vi "S4GUI.vi"(7 "Tab ObsEng":enum32{"Obs", "CCD modes", "Eng"}(tab)) -> ()   [LabVIEW 2018] (continued)
                    n457 = property on="setupCH4" class="Bool (strict)"("Blinking"=w1016) -> ()  [unwired: 2 in, 2 out]
                    n458 = property on="Disk Storage ch4" class="Slide (strict)"("Fill Color"=w1006) -> ()  [unwired: 2 in, 2 out]
                    n459 = Select(t=w1004, s=w1002, f=w1005) -> (s? t:f=w1003:cluster{u32, u32}[])
                    n460 = property on="Exposures Done ch4" class="Slide (strict)"("Caption.Text"=w1011) -> ()  [unwired: 2 in, 2 out]
                    n461 = property on="Channel 4" class="Bool (strict)"("Colors [4]"=w1003) -> ()  [unwired: 2 in, 2 out]
                    n462 = Number To Decimal String(number=w998) -> (decimal integer string=w1000:string)  [unwired: 1 in]
                    n463 = Concatenate Strings("Disk Storage ", w1000, "%" ("string")) -> (w997:string)
                    n464 = property on="Disk Storage ch4" class="Slide (strict)"("Caption.Text"=w997) -> ()  [unwired: 2 in, 2 out]
                  }
                }
              }
              frame #9 {
                n465 = Unbundle By Name(w1023) -> ("Instrument Status.mode"=w1022:bool)
                n466 = case shown="True" w1022 {
                  tunnel: [0 ("t") w1036] -> w1019
                  tunnel: w1023 -> [_ w1025]
                  frame False {
                    # "Fotometria: #PSD = 0"
                  }
                  frame True {
                    # "Polarimetria: calcula #PSD"
                    n467 = Unbundle By Name(w1025) -> ("WPROT seq"=w1029:u16)
                    n468 = Number To Boolean Array(number=w1029) -> (Boolean array=w1028:bool[])
                    n469 = for {
                      shift-right: [w1040] -> w1031
                      shift-left: 0 -> [w1038]
                      tunnel: w1028 -> [w1037] mode=indexing
                      # "calcula qtd de 1s"
                      n470 = Increment(x=w1038) -> (x+1=w1039:i32)
                      n471 = Select(t=w1039, s=w1037, f=w1038) -> (s? t:f=w1040:i32)
                    }
                    n472 = property on="#Pol. Seq. Done" class="Slide (strict)"() -> ("Scale.Maximum"=w1030:dbl)  [unwired: 2 in, 2 out]
                    n473 = To Long Integer(number=w1030) -> (32bit integer=w1032:i32)
                    n474 = Subtract(x=w1032, y=w1031) -> (x-y=w1033:i32)
                    n475 = Decrement(x=w1033) -> (x-1=w1035:i32)
                    n476 = Less Than 0?(x=w1035) -> (x < 0?=w1034:bool)
                    n477 = Select(t=0, s=w1034, f=w1035) -> (s? t:f=w1036:i32)
                  }
                }
                "#Pol. Seq. Done" <- w1019
                n478 = Number To Decimal String(number=w1019) -> (decimal integer string=w1020:string)  [unwired: 1 in]
                n479 = Concatenate Strings("#Pol. Seq. Done ", w1020) -> (w1018:string)
                n480 = property on="#Pol. Seq. Done" class="Slide (strict)"("Caption.Text"=w1018) -> ()  [unwired: 2 in, 2 out]
              }
              frame #10 {
                # "OVJ 2022-12-12: \nA visibilidade do Tab ObsEng sempre \nacompanha a habilitação do tab4."
                n481 = Unbundle By Name(w1050) -> ("Cluster ExpMode.tab4"=w1044:T12, "Cluster Polarimetry"=w1071:T22, "Cluster Mode Sync"=w1078:T23)
                n482 = case shown="\"Enabled\", Default" w1044 {
                  tunnel: [TRUE ("Tabs Visible?") w1080] -> w1049
                  frame "Enabled", Default {
                  }
                  frame "Disabled and Grayed Out" {
                    n483 = disable-structure shown="Enabled" {
                      disable-tunnel: [TRUE ("Tabs Visible?") FALSE ("Tabs Visible?")] -> w1080
                      frame Disabled {
                        # "DEBUG"
                      }
                      frame Enabled {
                      }
                    }
                  }
                }
                n484 = property on="Tab Acq Type" class="TabCtl (strict)"("DisabledEnum"=w1044) -> (error out=w1048:errorcluster)  [unwired: 2 in, 1 out]
                n485 = Unbundle By Name(w1078) -> ("Start SM Text"=w1077:string, "Star SM"=w1046:T12, "Pause SM"=w1076:T12, "Stop SM"=w1075:T12, "Abort SM"=w1074:T12, "#Cycles"=w1073:T12, "SSM"=w1072:T12, "Set SM"=w1041:T12, "#Index Cycles"=w1047:T12)
                n486 = property on="Observer" class="Str"(error in=w1048, "DisabledEnum"=w1044) -> (error out=w1043:errorcluster)  [unwired: 1 in, 1 out]
                n487 = property on="Tab ObsEng" class="TabCtl (strict)"("Tabs Visible?"=w1049) -> ()  [unwired: 2 in, 2 out]
                n488 = property on="Project ID" class="Str"(error in=w1043, "DisabledEnum"=w1044) -> (error out=w1042:errorcluster)  [unwired: 1 in, 1 out]
                n489 = property on="set keywords" class="Bool"(error in=w1042, "DisabledEnum"=w1041) -> (error out=w1045:errorcluster)  [unwired: 1 in, 1 out]
                n490 = property on="Start SM" class="Bool"("BoolText.Text"=w1077) -> ()  [unwired: 2 in, 2 out]
                n491 = property on="#Cycles Done" class="Slide (strict)"("DisabledEnum"=w1047) -> ()  [unwired: 2 in, 2 out]
                n492 = property on="Start SM" class="Bool"("DisabledEnum"=w1046) -> ()  [unwired: 2 in, 2 out]
                n493 = property on="Stop SM" class="Bool"("DisabledEnum"=w1075) -> ()  [unwired: 2 in, 2 out]
                n494 = property on="Abort SM" class="Bool"("DisabledEnum"=w1074) -> ()  [unwired: 2 in, 2 out]
                n495 = property on="Pause SM" class="Bool"("DisabledEnum"=w1076) -> ()  [unwired: 2 in, 2 out]
                n496 = property on="# Cycles" class="DigNum (strict)"("DisabledEnum"=w1073) -> ()  [unwired: 2 in, 2 out]
                n497 = property on="SSM" class="Ring (strict)"("DisabledEnum"=w1072) -> ()  [unwired: 2 in, 2 out]
                n498 = property on="set Observer" class="Bool"(error in=w1045, "DisabledEnum"=w1041) -> ()  [unwired: 1 in, 2 out]
                n499 = Unbundle By Name(w1071) -> ("Lambda Selector"=w1070:T12, "Calibrator Selector"=w1069:T12, "Set Waveplate"=w1068:T12, "Select Positions"=w1067:T12, "P0"=w1066:T12, "P8"=w1065:T12, "P1"=w1064:T12, "P9"=w1063:T12, "P2"=w1062:T12, "P10"=w1061:T12, "P3"=w1060:T12, "P11"=w1059:T12, "P4"=w1058:T12, "P12"=w1057:T12, "P5"=w1056:T12, "P13"=w1055:T12, "P6"=w1054:T12, "P14"=w1053:T12, "P7"=w1052:T12, "P15"=w1051:T12)
                n500 = property on="P0" class="Bool (strict)"("DisabledEnum"=w1066) -> ()  [unwired: 2 in, 2 out]
                n501 = property on="Lambda Selector" class="Ring (strict)"("DisabledEnum"=w1070) -> ()  [unwired: 2 in, 2 out]
                n502 = property on="Calibrator Selector" class="Ring (strict)"("DisabledEnum"=w1069) -> ()  [unwired: 2 in, 2 out]
                n503 = property on="Set Waveplate" class="Bool"("DisabledEnum"=w1068) -> ()  [unwired: 2 in, 2 out]
                n504 = property on="P1" class="Bool (strict)"("DisabledEnum"=w1064) -> ()  [unwired: 2 in, 2 out]
                n505 = property on="P2" class="Bool (strict)"("DisabledEnum"=w1062) -> ()  [unwired: 2 in, 2 out]
                n506 = property on="Select Positions" class="Ring (strict)"("DisabledEnum"=w1067) -> ()  [unwired: 2 in, 2 out]
                n507 = property on="P3" class="Bool (strict)"("DisabledEnum"=w1060) -> ()  [unwired: 2 in, 2 out]
                n508 = property on="P4" class="Bool (strict)"("DisabledEnum"=w1058) -> ()  [unwired: 2 in, 2 out]
                n509 = property on="P5" class="Bool (strict)"("DisabledEnum"=w1056) -> ()  [unwired: 2 in, 2 out]
                n510 = property on="P6" class="Bool (strict)"("DisabledEnum"=w1054) -> ()  [unwired: 2 in, 2 out]
                n511 = property on="P7" class="Bool (strict)"("DisabledEnum"=w1052) -> ()  [unwired: 2 in, 2 out]
                n512 = property on="P8" class="Bool (strict)"("DisabledEnum"=w1065) -> ()  [unwired: 2 in, 2 out]
                n513 = property on="P9" class="Bool (strict)"("DisabledEnum"=w1063) -> ()  [unwired: 2 in, 2 out]
                n514 = property on="P10" class="Bool (strict)"("DisabledEnum"=w1061) -> ()  [unwired: 2 in, 2 out]
                n515 = property on="P11" class="Bool (strict)"("DisabledEnum"=w1059) -> ()  [unwired: 2 in, 2 out]
                n516 = property on="P12" class="Bool (strict)"("DisabledEnum"=w1057) -> ()  [unwired: 2 in, 2 out]
                n517 = property on="P15" class="Bool (strict)"("DisabledEnum"=w1051) -> ()  [unwired: 2 in, 2 out]
                n518 = property on="P13" class="Bool (strict)"("DisabledEnum"=w1055) -> ()  [unwired: 2 in, 2 out]
                n519 = property on="P14" class="Bool (strict)"("DisabledEnum"=w1053) -> ()  [unwired: 2 in, 2 out]
              }
              frame #11 {
                n520 = Unbundle By Name(w1097) -> ("Cluster Mode CH1"=w1084:T24, "Cluster Mode Sync"=w1083:T23)
                n521 = Unbundle By Name(w1084) -> ("Start ch1 Text"=w1096:string, "#cycles ch1"=w1095:T12, "Start ch1"=w1094:T12, "Pause ch1"=w1093:T12, "Abort ch1"=w1092:T12, "Stop ch1"=w1091:T12, "Exptime ch1"=w1090:T12, "Exp ch1"=w1089:T12, "Set Cooler"=w1088:T12, "Set Temp"=w1087:T12)
                n522 = Unbundle By Name(w1083) -> ("#Index Cycles"=w1086:T12)
                n523 = case shown="Default" w1086 {
                  tunnel: [T12."Enabled" ("#Index Cycles") T12."Disabled and Grayed Out" ("#Index Cycles")] -> w1085
                  frame "Disabled and Grayed Out" {
                  }
                  frame Default {
                  }
                }
                n524 = property on="Start ch1" class="Bool"("BoolText.Text"=w1096) -> ()  [unwired: 2 in, 2 out]
                n525 = property on="Abort ch1" class="Bool"("DisabledEnum"=w1092) -> ()  [unwired: 2 in, 2 out]
                n526 = property on="Stop ch1" class="Bool"("DisabledEnum"=w1091) -> ()  [unwired: 2 in, 2 out]
                n527 = property on="#cycles ch1" class="DigNum (strict)"("DisabledEnum"=w1095) -> ()  [unwired: 2 in, 2 out]
                n528 = property on="Cooler 1" class="Bool (strict)"("DisabledEnum"=w1088) -> ()  [unwired: 2 in, 2 out]
                n529 = property on="Exptime ch1" class="DigNum (strict)"("DisabledEnum"=w1090) -> ()  [unwired: 2 in, 2 out]
                n530 = property on="Start ch1" class="Bool"("DisabledEnum"=w1094) -> ()  [unwired: 2 in, 2 out]
                n531 = property on="Set Temp 1" class="Bool"("DisabledEnum"=w1087) -> ()  [unwired: 2 in, 2 out]
                n532 = property on="Exp ch1" class="DigNum (strict)"("DisabledEnum"=w1089) -> ()  [unwired: 2 in, 2 out]
                n533 = property on="Cycles Done ch1" class="Slide (strict)"("DisabledEnum"=w1085) -> ()  [unwired: 2 in, 2 out]
                n534 = property on="Pause ch1" class="Bool"("DisabledEnum"=w1093) -> ()  [unwired: 2 in, 2 out]
              }
              frame #12 {
                n535 = Unbundle By Name(w1114) -> ("Cluster Mode CH2"=w1113:T25, "Cluster Mode Sync"=w1101:T23)
                n536 = Unbundle By Name(w1101) -> ("#Index Cycles"=w1102:T12)
                n537 = Unbundle By Name(w1113) -> ("Start ch2 Text"=w1112:string, "#cycles ch2"=w1111:T12, "Start ch2"=w1110:T12, "Pause ch2"=w1109:T12, "Stop ch2"=w1108:T12, "Abort ch2"=w1107:T12, "Exptime ch2"=w1106:T12, "Exp ch2"=w1105:T12, "Set Cooler"=w1104:T12, "Set Temp"=w1103:T12)
                n538 = case shown="\"Disabled and Grayed Out\"" w1102 {
                  tunnel: [T12."Enabled" ("#Index Cycles") T12."Disabled and Grayed Out" ("#Index Cycles")] -> w1100
                  frame "Disabled and Grayed Out" {
                  }
                  frame Default {
                  }
                }
                n539 = property on="Start ch2" class="Bool"("BoolText.Text"=w1112) -> ()  [unwired: 2 in, 2 out]
                n540 = property on="Stop ch2" class="Bool"("DisabledEnum"=w1108) -> ()  [unwired: 2 in, 2 out]
                n541 = property on="Abort ch2" class="Bool"("DisabledEnum"=w1107) -> ()  [unwired: 2 in, 2 out]
                n542 = property on="Cooler 2" class="Bool (strict)"("DisabledEnum"=w1104) -> ()  [unwired: 2 in, 2 out]
                n543 = property on="#cycles ch2" class="DigNum (strict)"("DisabledEnum"=w1111) -> ()  [unwired: 2 in, 2 out]
                n544 = property on="Exptime ch2" class="DigNum (strict)"("DisabledEnum"=w1106) -> ()  [unwired: 2 in, 2 out]
                n545 = property on="Set Temp 2" class="Bool"("DisabledEnum"=w1103) -> ()  [unwired: 2 in, 2 out]
                n546 = property on="Start ch2" class="Bool"("DisabledEnum"=w1110) -> ()  [unwired: 2 in, 2 out]
                n547 = property on="Cycles Done ch2" class="Slide (strict)"("DisabledEnum"=w1100) -> ()  [unwired: 2 in, 2 out]
                n548 = property on="Exp ch2" class="DigNum (strict)"("DisabledEnum"=w1105) -> ()  [unwired: 2 in, 2 out]
                n549 = property on="Pause ch2" class="Bool"("DisabledEnum"=w1109) -> ()  [unwired: 2 in, 2 out]
              }
              frame #13 {
                n550 = Unbundle By Name(w1131) -> ("Cluster Mode CH3"=w1130:T26, "Cluster Mode Sync"=w1118:T23)
                n551 = Unbundle By Name(w1118) -> ("#Index Cycles"=w1119:T12)
                n552 = Unbundle By Name(w1130) -> ("Start ch3 Text"=w1129:string, "#cycles ch3"=w1128:T12, "Start ch3"=w1127:T12, "Pause ch3"=w1126:T12, "Stop ch3"=w1125:T12, "Abort ch3"=w1124:T12, "Exptime ch3"=w1123:T12, "Exp ch3"=w1122:T12, "Set Cooler"=w1121:T12, "Set Temp"=w1120:T12)
                n553 = case shown="\"Disabled and Grayed Out\"" w1119 {
                  tunnel: [T12."Enabled" ("#Index Cycles") T12."Disabled and Grayed Out" ("#Index Cycles")] -> w1117
                  frame "Disabled and Grayed Out" {
                  }
                  frame Default {
                  }
                }
                n554 = property on="Start ch3" class="Bool"("BoolText.Text"=w1129) -> ()  [unwired: 2 in, 2 out]
                n555 = property on="Stop ch3" class="Bool"("DisabledEnum"=w1125) -> ()  [unwired: 2 in, 2 out]
                n556 = property on="Abort ch3" class="Bool"("DisabledEnum"=w1124) -> ()  [unwired: 2 in, 2 out]
                n557 = property on="Cycles Done ch3" class="Slide (strict)"("DisabledEnum"=w1117) -> ()  [unwired: 2 in, 2 out]
                n558 = property on="Cooler 3" class="Bool (strict)"("DisabledEnum"=w1121) -> ()  [unwired: 2 in, 2 out]
                n559 = property on="#cycles ch3" class="DigNum (strict)"("DisabledEnum"=w1128) -> ()  [unwired: 2 in, 2 out]
                n560 = property on="Set Temp 3" class="Bool"("DisabledEnum"=w1120) -> ()  [unwired: 2 in, 2 out]
                n561 = property on="Exptime ch3" class="DigNum (strict)"("DisabledEnum"=w1123) -> ()  [unwired: 2 in, 2 out]
                n562 = property on="Start ch3" class="Bool"("DisabledEnum"=w1127) -> ()  [unwired: 2 in, 2 out]
                n563 = property on="Exp ch3" class="DigNum (strict)"("DisabledEnum"=w1122) -> ()  [unwired: 2 in, 2 out]
                n564 = property on="Pause ch3" class="Bool"("DisabledEnum"=w1126) -> ()  [unwired: 2 in, 2 out]
              }
              frame #14 {
                n565 = Unbundle By Name(w1148) -> ("Cluster Mode CH4"=w1147:T27, "Cluster Mode Sync"=w1135:T23)
                n566 = Unbundle By Name(w1135) -> ("#Index Cycles"=w1136:T12)
                n567 = Unbundle By Name(w1147) -> ("Start ch4 Text"=w1146:string, "#cycles ch4"=w1145:T12, "Start ch4"=w1144:T12, "Pause ch4"=w1143:T12, "Stop ch4"=w1142:T12, "Abort ch4"=w1141:T12, "Exptime ch4"=w1140:T12, "Exp ch4"=w1139:T12, "Set Cooler"=w1138:T12, "Set Temp"=w1137:T12)
                n568 = case shown="\"Disabled and Grayed Out\"" w1136 {
                  tunnel: [T12."Enabled" ("#Index Cycles") T12."Disabled and Grayed Out" ("#Index Cycles")] -> w1134
                  frame "Disabled and Grayed Out" {
                  }
                  frame Default {
                  }
                }
                n569 = property on="Start ch4" class="Bool"("BoolText.Text"=w1146) -> ()  [unwired: 2 in, 2 out]
                n570 = property on="Stop ch4" class="Bool"("DisabledEnum"=w1142) -> ()  [unwired: 2 in, 2 out]
                n571 = property on="Cooler 4" class="Bool (strict)"("DisabledEnum"=w1138) -> ()  [unwired: 2 in, 2 out]
                n572 = property on="Set Temp 4" class="Bool"("DisabledEnum"=w1137) -> ()  [unwired: 2 in, 2 out]
                n573 = property on="Abort ch4" class="Bool"("DisabledEnum"=w1141) -> ()  [unwired: 2 in, 2 out]
                n574 = property on="#cycles ch4" class="DigNum (strict)"("DisabledEnum"=w1145) -> ()  [unwired: 2 in, 2 out]
                n575 = property on="Exptime ch4" class="DigNum (strict)"("DisabledEnum"=w1140) -> ()  [unwired: 2 in, 2 out]
                n576 = property on="Cycles Done ch4" class="Slide (strict)"("DisabledEnum"=w1134) -> ()  [unwired: 2 in, 2 out]
                n577 = property on="Start ch4" class="Bool"("DisabledEnum"=w1144) -> ()  [unwired: 2 in, 2 out]
                n578 = property on="Exp ch4" class="DigNum (strict)"("DisabledEnum"=w1139) -> ()  [unwired: 2 in, 2 out]
                n579 = property on="Pause ch4" class="Bool"("DisabledEnum"=w1143) -> ()  [unwired: 2 in, 2 out]
              }
              frame #15 {
                # "Carrega coluna do Channel 1"
                # "Aba:  Eng->Camera"
                n580 = Unbundle By Name(w1215) -> ("ChannelA_CCD"=w1160:T28, "CHA_Checked Params"=w1206:T14, "ChannelA_Status.connection"=w1159:bool)
                n581 = Unbundle By Name(w1206) -> ("ACQUISITION_MODE"=w1184:bool, "TRIGGER_MODE"=w1185:bool, "READ_MODE"=w1186:bool, "PREAMP"=w1194:bool, "READOUT_RATE"=w1195:bool, "VERTICAL_SHIFT_SPEED"=w1196:bool, "EM_MODE"=w1197:bool, "EM_GAIN"=w1187:bool, "SHUTTER_MODE"=w1188:bool, "SHUTTER_TTL"=w1189:bool, "SHUTTER_OPENING_TIME"=w1190:bool, "SHUTTER_CLOSING_TIME"=w1191:bool, "VBIN"=w1192:bool, "HBIN"=w1193:bool, "INITIAL_LINE"=w1198:bool, "INITIAL_COLUMN"=w1203:bool, "FINAL_LINE"=w1205:bool, "FINAL_COLUMN"=w1202:bool, "FRAME_TRANSFER"=w1201:bool, "VERTICAL_CLOCK_VOLTAGE"=w1200:bool, "AD_CHANNEL"=w1199:bool)
                n582 = local read "CH1on"() -> (w1152:bool)
                n583 = Unbundle By Name(w1160) -> ("INITIAL_LINE"=w1182:u16, "INITIAL_COLUMN"=w1181:u16, "FINAL_LINE"=w1180:u16, "FINAL_COLUMN"=w1179:u16, "VBIN"=w1178:u16, "HBIN"=w1177:u16, "PREAMP"=w1176:u8, "EM_GAIN"=w1175:u16, "READOUT_RATE"=w1174:u8, "SHUTTER_OPENNING_TIME"=w1173:u16, "SHUTTER_CLOSING_TIME"=w1172:u16, "VERTICAL_SHIFT_SPEED"=w1171:u8, "READ_MODE"=w1170:u8, "VERTICAL_CLOCK_VOLTAGE"=w1169:u8, "AD_CHANNEL"=w1168:u32, "SHUTTER_MODE"=w1167:u8, "SHUTTER_TTL"=w1166:u8, "TRIGGER_MODE"=w1165:u8, "FRAME_TRANSFER"=w1164:bool, "ACQUISITION_MODE"=w1162:u8, "EM_MODE"=w1161:u8)
                n584 = Equal?(x=w1210, y="none") -> (x = y?=w1207:bool)
                n585 = Equal?(x=w1210, y="default.cfg") -> (x = y?=w1208:bool)
                n586 = Or(x=w1208, y=w1207) -> (x .or. y?=w1209:bool)
                n587 = case shown="True" w1209 {
                  tunnel: [T12."Enabled" ("Disabled") T12."Disabled and Grayed Out" ("Disabled")] -> w1212
                  frame False {
                    # "Se Curr Conf File != default.cfg,\nhabilita botão de Salvar."
                  }
                  frame True {
                    # "Não é permitido salvar em \ncima de default.cfg"
                  }
                }
                n588 = case shown="True" w1159 {
                  tunnel: w1160 -> [_ w1268]
                  tunnel: [w1261 w1267] -> w1158
                  tunnel: [w1261 w1266] -> w1157
                  tunnel: [w1261 w1265] -> w1156
                  tunnel: [w1261 w1264] -> w1155
                  tunnel: [w1261 w1263] -> w1154
                  tunnel: [w1261 w1262] -> w1153
                  frame False {
                    w1261 = "" ("RO1")
                  }
                  frame True {
                    n589 = stacked-sequence "Atualizacao dos indicadores inferiores do CANAL A da tela principal" {
                      tunnel: w1268 -> [w1283 w1286 w1291 w1300 w1303 w1307]
                      tunnel: [w1269 _ _ _ _ _] -> w1267
                      tunnel: [_ w1284 _ _ _ _] -> w1266
                      tunnel: [_ _ w1289 _ _ _] -> w1265
                      tunnel: [_ _ _ w1294 _ _] -> w1264
                      tunnel: [_ _ _ _ w1301 _] -> w1263
                      tunnel: [_ _ _ _ _ w1304] -> w1262
                      frame #0 {
                        # "SubImage"
                        n590 = Unbundle By Name(w1283) -> ("INITIAL_LINE"=w1281:u16, "FINAL_LINE"=w1280:u16, "INITIAL_COLUMN"=w1279:u16, "FINAL_COLUMN"=w1278:u16)
                        n591 = Number To Decimal String(number=w1281) -> (decimal integer string=w1277:string)  [unwired: 1 in]
                        n592 = Number To Decimal String(number=w1280) -> (decimal integer string=w1275:string)  [unwired: 1 in]
                        n593 = Number To Decimal String(number=w1279) -> (decimal integer string=w1273:string)  [unwired: 1 in]
                        n594 = Number To Decimal String(number=w1278) -> (decimal integer string=w1271:string)  [unwired: 1 in]
                        n595 = Concatenate Strings("[", w1277, ":", w1275, ",", w1273, ":", w1271, "]") -> (w1269:string)
                      }
                      frame #1 {
                        # "Em Active"
                        n596 = Unbundle By Name(w1286) -> ("EM_MODE"=w1285:u8)
                        n597 = case shown="0, Default" w1285 {
                          tunnel: ["Electron M." ("EmActive1") "Convent." ("EmActive1")] -> w1284
                          frame 0, Default {
                          }
                          frame 1 {
                          }
                        }
                      }
                      frame #2 {
                        # "Pre Amp"
                        n598 = Unbundle By Name(w1291) -> ("PREAMP"=w1290:u8)
                        n599 = case shown="1" w1290 {
                          tunnel: ["Gain 1" ("EmActive1") "Gain 2" ("EmActive1")] -> w1289
                          frame 0, Default {
                          }
                          frame 1 {
                          }
                        }
                      }
                      frame #3 {
                        # "Binning"
                        n600 = Unbundle By Name(w1300) -> ("VBIN"=w1299:u16, "HBIN"=w1298:u16)
                        n601 = Number To Decimal String(number=w1298) -> (decimal integer string=w1295:string)  [unwired: 1 in]
                        n602 = Number To Decimal String(number=w1299) -> (decimal integer string=w1297:string)  [unwired: 1 in]
                        n603 = Concatenate Strings(w1297, "x", w1295) -> (w1294:string)
                      }
                      frame #4 {
                        # "Gain"
                        n604 = Unbundle By Name(w1303) -> ("EM_GAIN"=w1302:u16)
                        n605 = Number To Decimal String(number=w1302) -> (decimal integer string=w1301:string)  [unwired: 1 in]
                      }
                      frame #5 {
                        # "Readout"
                        n606 = Unbundle By Name(w1307) -> ("EM_MODE"=w1306:u8, "READOUT_RATE"=w1305:u8)
                        n607 = case shown="0, Default" w1306 {
                          tunnel: w1305 -> [w1309 w1315]
                          tunnel: [w1308 w1314] -> w1304
                          frame 0, Default {
                            n608 = case shown="0, Default" w1309 {
                              tunnel: ["30 MHz" ("EmActive1") "20 MHz" ("EmActive1") "10 MHz" ("EmActive1") "1 MHz" ("EmActive1")] -> w1308
                              frame 0, Default {
                              }
                              frame 1 {
                              }
                              frame 2 {
                              }
                              frame 3 {
                              }
                            }
                          }
                          frame 1 {
                            n609 = case shown="1" w1315 {
                              tunnel: ["1 MHz" ("EmActive1") "0.1 MHz" ("EmActive1")] -> w1314
                              frame 0, Default {
                              }
                              frame 1 {
                              }
                            }
                          }
                        }
                      }
                    }
                  }
                }
                n610 = case shown="False" w1152 {
                  tunnel: w1205 -> [_ w1260]
                  tunnel: w1203 -> [_ w1256]
                  tunnel: w1202 -> [_ w1254]
                  tunnel: w1201 -> [_ w1250]
                  tunnel: w1200 -> [_ w1249]
                  tunnel: w1199 -> [_ w1248]
                  tunnel: w1198 -> [_ w1240]
                  tunnel: w1197 -> [_ w1232]
                  tunnel: w1196 -> [_ w1231]
                  tunnel: w1195 -> [_ w1230]
                  tunnel: w1194 -> [_ w1229]
                  tunnel: w1193 -> [_ w1228]
                  tunnel: w1192 -> [_ w1227]
                  tunnel: w1191 -> [_ w1226]
                  tunnel: w1190 -> [_ w1225]
                  tunnel: w1189 -> [_ w1224]
                  tunnel: w1188 -> [_ w1223]
                  tunnel: w1187 -> [_ w1222]
                  tunnel: w1186 -> [_ w1221]
                  tunnel: w1185 -> [_ w1220]
                  tunnel: w1184 -> [_ w1219]
                  tunnel: [T12."Disabled and Grayed Out" ("Disabled") T12."Enabled" ("Disabled")] -> w1151
                  frame False {
                    w1216 = FALSE
                    n611 = property on="Image FInal Column" class="DigNum (strict)"("Blinking"=w1216) -> ()  [unwired: 2 in, 2 out]
                    n612 = property on="Frame Transfer" class="Bool (strict)"("Blinking"=w1216) -> ()  [unwired: 2 in, 2 out]
                    n613 = property on="Vertical Clock Voltage" class="Ring (strict)"("Blinking"=w1216) -> ()  [unwired: 2 in, 2 out]
                    n614 = property on="A/D  Channel" class="DigNum (strict)"("Blinking"=w1216) -> ()  [unwired: 2 in, 2 out]
                    n615 = property on="Image Initial Line" class="DigNum (strict)"("Blinking"=w1216) -> ()  [unwired: 2 in, 2 out]
                    n616 = property on="Image Initial Column" class="DigNum (strict)"("Blinking"=w1216) -> ()  [unwired: 2 in, 2 out]
                    n617 = property on="Image Final Line" class="DigNum (strict)"("Blinking"=w1216) -> ()  [unwired: 2 in, 2 out]
                    n618 = property on="Shutter Openning Time" class="DigNum (strict)"("Blinking"=w1216) -> ()  [unwired: 2 in, 2 out]
                    n619 = property on="Shutter Closing Time" class="DigNum (strict)"("Blinking"=w1216) -> ()  [unwired: 2 in, 2 out]
                    n620 = property on="Vertical Binning" class="DigNum (strict)"("Blinking"=w1216) -> ()  [unwired: 2 in, 2 out]
                    n621 = property on="Horizontal Binning" class="DigNum (strict)"("Blinking"=w1216) -> ()  [unwired: 2 in, 2 out]
                    n622 = property on="CCD EM Gain" class="DigNum (strict)"("Blinking"=w1216) -> ()  [unwired: 2 in, 2 out]
                    n623 = property on="Shutter Mode" class="Ring (strict)"("Blinking"=w1216) -> ()  [unwired: 2 in, 2 out]
                    n624 = property on="Shutter TTL" class="Ring (strict)"("Blinking"=w1216) -> ()  [unwired: 2 in, 2 out]
                    n625 = property on="Acquisition Mode" class="Ring (strict)"("Blinking"=w1216) -> ()  [unwired: 2 in, 2 out]
                    n626 = property on="Readout Rate" class="Ring (strict)"("Blinking"=w1216) -> ()  [unwired: 2 in, 2 out]
                    n627 = property on="Vertical Shift Speed" class="Ring (strict)"("Blinking"=w1216) -> ()  [unwired: 2 in, 2 out]
                    n628 = property on="CCD EM Mode" class="Ring (strict)"("Blinking"=w1216) -> ()  [unwired: 2 in, 2 out]
                    n629 = property on="Trigger Mode" class="Ring (strict)"("Blinking"=w1216) -> ()  [unwired: 2 in, 2 out]
                    n630 = property on="Read Mode" class="Ring (strict)"("Blinking"=w1216) -> ()  [unwired: 2 in, 2 out]
                    n631 = property on="Pre-amplification Gain" class="Ring (strict)"("Blinking"=w1216) -> ()  [unwired: 2 in, 2 out]
                  }
                  frame True {
                    n632 = Not(x=w1254) -> (.not. x?=w1255:bool)
                    n633 = Not(x=w1250) -> (.not. x?=w1252:bool)
                    n634 = Not(x=w1249) -> (.not. x?=w1253:bool)
                    n635 = Not(x=w1248) -> (.not. x?=w1251:bool)
                    n636 = Not(x=w1240) -> (.not. x?=w1258:bool)
                    n637 = Not(x=w1256) -> (.not. x?=w1257:bool)
                    n638 = Not(x=w1260) -> (.not. x?=w1259:bool)
                    n639 = property on="Image FInal Column" class="DigNum (strict)"("Blinking"=w1255) -> ()  [unwired: 2 in, 2 out]
                    n640 = property on="Frame Transfer" class="Bool (strict)"("Blinking"=w1252) -> ()  [unwired: 2 in, 2 out]
                    n641 = property on="Vertical Clock Voltage" class="Ring (strict)"("Blinking"=w1253) -> ()  [unwired: 2 in, 2 out]
                    n642 = property on="A/D  Channel" class="DigNum (strict)"("Blinking"=w1251) -> ()  [unwired: 2 in, 2 out]
                    n643 = property on="Image Initial Line" class="DigNum (strict)"("Blinking"=w1258) -> ()  [unwired: 2 in, 2 out]
                    n644 = property on="Image Initial Column" class="DigNum (strict)"("Blinking"=w1257) -> ()  [unwired: 2 in, 2 out]
                    n645 = property on="Image Final Line" class="DigNum (strict)"("Blinking"=w1259) -> ()  [unwired: 2 in, 2 out]
                    n646 = Not(x=w1225) -> (.not. x?=w1244:bool)
                    n647 = Not(x=w1226) -> (.not. x?=w1246:bool)
                    n648 = Not(x=w1227) -> (.not. x?=w1245:bool)
                    n649 = Not(x=w1228) -> (.not. x?=w1247:bool)
                    n650 = Not(x=w1222) -> (.not. x?=w1242:bool)
                    n651 = Not(x=w1223) -> (.not. x?=w1243:bool)
                    n652 = Not(x=w1224) -> (.not. x?=w1241:bool)
                    n653 = property on="Shutter Openning Time" class="DigNum (strict)"("Blinking"=w1244) -> ()  [unwired: 2 in, 2 out]
                    n654 = property on="Shutter Closing Time" class="DigNum (strict)"("Blinking"=w1246) -> ()  [unwired: 2 in, 2 out]
                    n655 = property on="Vertical Binning" class="DigNum (strict)"("Blinking"=w1245) -> ()  [unwired: 2 in, 2 out]
                    n656 = property on="Horizontal Binning" class="DigNum (strict)"("Blinking"=w1247) -> ()  [unwired: 2 in, 2 out]
                    n657 = property on="CCD EM Gain" class="DigNum (strict)"("Blinking"=w1242) -> ()  [unwired: 2 in, 2 out]
                    n658 = property on="Shutter Mode" class="Ring (strict)"("Blinking"=w1243) -> ()  [unwired: 2 in, 2 out]
                    n659 = property on="Shutter TTL" class="Ring (strict)"("Blinking"=w1241) -> ()  [unwired: 2 in, 2 out]
                    n660 = Not(x=w1219) -> (.not. x?=w1233:bool)
                    n661 = Not(x=w1230) -> (.not. x?=w1236:bool)
                    n662 = Not(x=w1231) -> (.not. x?=w1234:bool)
                    n663 = Not(x=w1232) -> (.not. x?=w1235:bool)
                    n664 = Not(x=w1220) -> (.not. x?=w1238:bool)
                    n665 = Not(x=w1221) -> (.not. x?=w1237:bool)
                    n666 = Not(x=w1229) -> (.not. x?=w1239:bool)
                    n667 = property on="Acquisition Mode" class="Ring (strict)"("Blinking"=w1233) -> ()  [unwired: 2 in, 2 out]
                    n668 = property on="Readout Rate" class="Ring (strict)"("Blinking"=w1236) -> ()  [unwired: 2 in, 2 out]
                    n669 = property on="Vertical Shift Speed" class="Ring (strict)"("Blinking"=w1234) -> ()  [unwired: 2 in, 2 out]
                    n670 = property on="CCD EM Mode" class="Ring (strict)"("Blinking"=w1235) -> ()  [unwired: 2 in, 2 out]
                    n671 = property on="Trigger Mode" class="Ring (strict)"("Blinking"=w1238) -> ()  [unwired: 2 in, 2 out]
                    n672 = property on="Read Mode" class="Ring (strict)"("Blinking"=w1237) -> ()  [unwired: 2 in, 2 out]
                    n673 = property on="Pre-amplification Gain" class="Ring (strict)"("Blinking"=w1239) -> ()  [unwired: 2 in, 2 out]
                  }
                }
                n674 = property on="Save Button" class="Bool (strict)"("DisabledEnum"=w1212) -> ()  [unwired: 2 in, 2 out]
                n675 = First Call?() -> (First Call?: T/F=w1183:bool)
                n676 = case shown="True" w1183 {
                  tunnel: w1182 -> [_ w1338]
                  tunnel: w1181 -> [_ w1337]
                  tunnel: w1180 -> [_ w1336]
                  tunnel: w1179 -> [_ w1335]
                  tunnel: w1178 -> [_ w1334]
                  tunnel: w1177 -> [_ w1333]
                  tunnel: w1176 -> [_ w1332]
                  tunnel: w1175 -> [_ w1331]
                  tunnel: w1174 -> [_ w1330]
                  tunnel: w1173 -> [_ w1329]
                  tunnel: w1172 -> [_ w1328]
                  tunnel: w1171 -> [_ w1327]
                  tunnel: w1170 -> [_ w1326]
                  tunnel: w1169 -> [_ w1325]
                  tunnel: w1168 -> [_ w1324]
                  tunnel: w1167 -> [_ w1323]
                  tunnel: w1166 -> [_ w1322]
                  tunnel: w1165 -> [_ w1321]
                  tunnel: w1164 -> [_ w1320]
                  tunnel: w1162 -> [_ w1319]
                  tunnel: w1161 -> [_ w1318]
                  frame False {
                  }
                  frame True {
                    n677 = local read "Input Cluster"() -> (w1342:T8)
                    n678 = Unbundle By Name(w1342) -> ("Parameters"=w1340:T5)
                    n679 = Bundle By Name(cluster=w1340, "Image \nInitial Line"=w1338, "Image\nInitial Column"=w1337, "Image\nFinal Line"=w1336, "Image\nFInal Column"=w1335, "Vertical\nBinning"=w1334, "Horizontal\nBinning"=w1333, "Pre-amplification\nGain"=w1332, "CCD\nEM Gain"=w1331, "Readout\nRate"=w1330, "Shutter\nOpenning Time"=w1329, "Shutter\nClosing Time"=w1328, "Vertical\nShift Speed"=w1327, "Read\nMode"=w1326, "Vertical\nClock Voltage"=w1325, "A/D \nChannel"=w1324, "Shutter\nMode"=w1323, "Shutter\nTTL"=w1322, "Trigger\nMode"=w1321, "Frame\nTransfer"=w1320, "Acquisition\nMode"=w1319, "CCD \nEM Mode"=w1318) -> (w1339:T5)
                    n680 = Bundle By Name(cluster=w1342, "Parameters"=w1339) -> (w1341:T8)
                    n681 = local write "Input Cluster"(w1341) -> ()
                  }
                }
                n682 = local read "Cameras Cluster"() -> (w1214:T7)
                n683 = Bundle By Name(cluster=w1214, "Current Configuration.Image Initial Line"=w1182, "Current Configuration.Image Initial Column"=w1181, "Current Configuration.Image Final Line"=w1180, "Current Configuration.Image FInal Column"=w1179, "Current Configuration.Vertical Binning"=w1178, "Current Configuration.Horizontal Binning"=w1177, "Current Configuration.Pre-amplification Gain"=w1176, "Current Configuration.CCD EM Gain"=w1175, "Current Configuration.Readout Rate"=w1174, "Current Configuration.Shutter Openning Time"=w1173, "Current Configuration.Shutter Closing Time"=w1172, "Current Configuration.Vertical Shift Speed"=w1171, "Current Configuration.Read Mode"=w1170, "Current Configuration.Vertical Clock Voltage"=w1169, "Current Configuration.A/D  Channel"=w1168, "Current Configuration.Shutter Mode"=w1167, "Current Configuration.Shutter TTL"=w1166, "Current Configuration.Trigger Mode"=w1165, "Current Configuration.Frame Transfer"=w1164, "Current Configuration.Acquisition Mode"=w1162, "Current Configuration.CCD EM Mode"=w1161) -> (w1163:T7)
                n684 = local write "RO1"(w1153) -> ()
                n685 = local write "SI1"(w1158) -> ()
                n686 = local write "EA1"(w1157) -> ()
                n687 = local write "PA1"(w1156) -> ()
                n688 = local write "B1"(w1155) -> ()
                n689 = local write "G1"(w1154) -> ()
                n690 = local write "Cameras Cluster"(w1163) -> ()
                n691 = Compound Arithmetic op=AND(w1184, w1185, w1186, w1194, w1195, w1196, w1197, w1187, w1188, w1189, w1190, w1191, w1192, w1193, w1198, w1203, w1205, w1202, w1201, w1200, w1199) -> (→"CCD checked 1":bool)
                n692 = property on="Shutter Openning Time" class="DigNum (strict)"("DisabledEnum"=w1151) -> ()  [unwired: 2 in, 2 out]
                n693 = property on="Shutter Closing Time" class="DigNum (strict)"("DisabledEnum"=w1151) -> ()  [unwired: 2 in, 2 out]
                n694 = property on="Vertical Binning" class="DigNum (strict)"("DisabledEnum"=w1151) -> ()  [unwired: 2 in, 2 out]
                n695 = property on="Horizontal Binning" class="DigNum (strict)"("DisabledEnum"=w1151) -> ()  [unwired: 2 in, 2 out]
                n696 = property on="CCD EM Gain" class="DigNum (strict)"("DisabledEnum"=w1151) -> ()  [unwired: 2 in, 2 out]
                n697 = property on="Shutter Mode" class="Ring (strict)"("DisabledEnum"=w1151) -> ()  [unwired: 2 in, 2 out]
                n698 = property on="Shutter TTL" class="Ring (strict)"("DisabledEnum"=w1151) -> ()  [unwired: 2 in, 2 out]
                n699 = property on="Acquisition Mode" class="Ring (strict)"("DisabledEnum"=w1151) -> ()  [unwired: 2 in, 2 out]
                n700 = property on="Readout Rate" class="Ring (strict)"("DisabledEnum"=w1151) -> ()  [unwired: 2 in, 2 out]
                n701 = property on="Vertical Shift Speed" class="Ring (strict)"("DisabledEnum"=w1151) -> ()  [unwired: 2 in, 2 out]
                n702 = property on="CCD EM Mode" class="Ring (strict)"("DisabledEnum"=w1151) -> ()  [unwired: 2 in, 2 out]
                n703 = property on="Trigger Mode" class="Ring (strict)"("DisabledEnum"=w1151) -> ()  [unwired: 2 in, 2 out]
                n704 = property on="Read Mode" class="Ring (strict)"("DisabledEnum"=w1151) -> ()  [unwired: 2 in, 2 out]
                n705 = property on="Pre-amplification Gain" class="Ring (strict)"("DisabledEnum"=w1151) -> ()  [unwired: 2 in, 2 out]
                n706 = property on="Image FInal Column" class="DigNum (strict)"("DisabledEnum"=w1151) -> ()  [unwired: 2 in, 2 out]
                n707 = property on="Frame Transfer" class="Bool (strict)"("DisabledEnum"=w1151) -> ()  [unwired: 2 in, 2 out]
                n708 = property on="Vertical Clock Voltage" class="Ring (strict)"("DisabledEnum"=w1151) -> ()  [unwired: 2 in, 2 out]
                n709 = property on="A/D  Channel" class="DigNum (strict)"("DisabledEnum"=w1151) -> ()  [unwired: 2 in, 2 out]
                n710 = property on="Image Initial Line" class="DigNum (strict)"("DisabledEnum"=w1151) -> ()  [unwired: 2 in, 2 out]
                n711 = property on="Image Initial Column" class="DigNum (strict)"("DisabledEnum"=w1151) -> ()  [unwired: 2 in, 2 out]
                n712 = property on="Image Final Line" class="DigNum (strict)"("DisabledEnum"=w1151) -> ()  [unwired: 2 in, 2 out]
                "Current Configuration File:" <- w1210
              }
              frame #16 {
                # "Carrega coluna do Channel 2"
                # "Aba:  Eng->Camera"
                n713 = Unbundle By Name(w1401) -> ("ChannelB_CCD"=w1357:T28, "CHB_Checked Params"=w1358:T14, "ChannelB_Status.connection"=w1356:bool)
                n714 = Unbundle By Name(w1358) -> ("ACQUISITION_MODE"=w1374:bool, "TRIGGER_MODE"=w1373:bool, "READ_MODE"=w1372:bool, "PREAMP"=w1371:bool, "READOUT_RATE"=w1347:bool, "VERTICAL_SHIFT_SPEED"=w1346:bool, "EM_MODE"=w1370:bool, "EM_GAIN"=w1381:bool, "SHUTTER_MODE"=w1380:bool, "SHUTTER_TTL"=w1379:bool, "SHUTTER_OPENING_TIME"=w1378:bool, "SHUTTER_CLOSING_TIME"=w1377:bool, "VBIN"=w1376:bool, "HBIN"=w1375:bool, "INITIAL_LINE"=w1388:bool, "INITIAL_COLUMN"=w1387:bool, "FINAL_LINE"=w1386:bool, "FINAL_COLUMN"=w1385:bool, "FRAME_TRANSFER"=w1384:bool, "VERTICAL_CLOCK_VOLTAGE"=w1383:bool, "AD_CHANNEL"=w1382:bool)
                n715 = case shown="True" w1356 {
                  tunnel: w1357 -> [_ w1458]
                  tunnel: [w1451 w1457] -> w1355
                  tunnel: [w1451 w1456] -> w1354
                  tunnel: [w1451 w1455] -> w1353
                  tunnel: [w1451 w1454] -> w1352
                  tunnel: [w1451 w1453] -> w1351
                  tunnel: [w1451 w1452] -> w1350
                  frame False {
                    w1451 = "" ("EmActive1")
                  }
                  frame True {
                    n716 = stacked-sequence "Atualizacao dos indicadores inferiores do CANAL B da tela principal" {
                      tunnel: w1458 -> [w1473 w1476 w1481 w1490 w1493 w1497]
                      tunnel: [_ w1474 _ _ _ _] -> w1457
                      tunnel: [_ _ w1479 _ _ _] -> w1456
                      tunnel: [_ _ _ w1484 _ _] -> w1455
                      tunnel: [_ _ _ _ w1491 _] -> w1454
                      tunnel: [_ _ _ _ _ w1494] -> w1453
                      tunnel: [w1459 _ _ _ _ _] -> w1452
                      frame #0 {
                        # "SubImage"
                        n717 = Unbundle By Name(w1473) -> ("INITIAL_LINE"=w1471:u16, "FINAL_LINE"=w1470:u16, "INITIAL_COLUMN"=w1469:u16, "FINAL_COLUMN"=w1468:u16)
                        n718 = Number To Decimal String(number=w1471) -> (decimal integer string=w1467:string)  [unwired: 1 in]
                        n719 = Number To Decimal String(number=w1470) -> (decimal integer string=w1465:string)  [unwired: 1 in]
                        n720 = Number To Decimal String(number=w1469) -> (decimal integer string=w1463:string)  [unwired: 1 in]
                        n721 = Number To Decimal String(number=w1468) -> (decimal integer string=w1461:string)  [unwired: 1 in]
                        n722 = Concatenate Strings("[", w1467, ":", w1465, ",", w1463, ":", w1461, "]") -> (w1459:string)
                      }
                      frame #1 {
                        # "Em Active"
                        n723 = Unbundle By Name(w1476) -> ("EM_MODE"=w1475:u8)
                        n724 = case shown="0, Default" w1475 {
                          tunnel: ["Electron M." ("EmActive1") "Convent." ("EmActive1")] -> w1474
                          frame 0, Default {
                          }
                          frame 1 {
                          }
                        }
                      }
                      frame #2 {
                        # "Pre Amp"
                        n725 = Unbundle By Name(w1481) -> ("PREAMP"=w1480:u8)
                        n726 = case shown="1" w1480 {
                          tunnel: ["Gain 1" ("EmActive1") "Gain 2" ("EmActive1")] -> w1479
                          frame 0, Default {
                          }
                          frame 1 {
                          }
                        }
                      }
                      frame #3 {
                        # "Binning"
                        n727 = Unbundle By Name(w1490) -> ("VBIN"=w1489:u16, "HBIN"=w1488:u16)
                        n728 = Number To Decimal String(number=w1488) -> (decimal integer string=w1486:string)  [unwired: 1 in]
                        n729 = Number To Decimal String(number=w1489) -> (decimal integer string=w1487:string)  [unwired: 1 in]
                        n730 = Concatenate Strings(w1487, "x", w1486) -> (w1484:string)
                      }
                      frame #4 {
                        # "Gain"
                        n731 = Unbundle By Name(w1493) -> ("EM_GAIN"=w1492:u16)
                        n732 = Number To Decimal String(number=w1492) -> (decimal integer string=w1491:string)  [unwired: 1 in]
                      }
                      frame #5 {
                        # "Readout"
                        n733 = Unbundle By Name(w1497) -> ("EM_MODE"=w1496:u8, "READOUT_RATE"=w1495:u8)
                        n734 = case shown="0, Default" w1496 {
                          tunnel: w1495 -> [w1499 w1505]
                          tunnel: [w1498 w1504] -> w1494
                          frame 0, Default {
                            n735 = case shown="3" w1499 {
                              tunnel: ["30 MHz" ("EmActive1") "20 MHz" ("EmActive1") "10 MHz" ("EmActive1") "1 MHz" ("EmActive1")] -> w1498
                              frame 0, Default {
                              }
                              frame 1 {
                              }
                              frame 2 {
                              }
                              frame 3 {
                              }
                            }
                          }
                          frame 1 {
                            n736 = case shown="1" w1505 {
                              tunnel: ["1 MHz" ("EmActive1") "0.1 MHz" ("EmActive1")] -> w1504
                              frame 0, Default {
                              }
                              frame 1 {
                              }
                            }
                          }
                        }
                      }
                    }
                  }
                }
                n737 = Unbundle By Name(w1357) -> ("INITIAL_LINE"=w1363:u16, "INITIAL_COLUMN"=w1361:u16, "FINAL_LINE"=w1364:u16, "FINAL_COLUMN"=w1362:u16, "VBIN"=w1367:u16, "HBIN"=w1398:u16, "PREAMP"=w1366:u8, "EM_GAIN"=w1365:u16, "READOUT_RATE"=w1360:u8, "SHUTTER_OPENNING_TIME"=w1397:u16, "SHUTTER_CLOSING_TIME"=w1396:u16, "VERTICAL_SHIFT_SPEED"=w1395:u8, "READ_MODE"=w1394:u8, "VERTICAL_CLOCK_VOLTAGE"=w1393:u8, "AD_CHANNEL"=w1392:u32, "SHUTTER_MODE"=w1389:u8, "SHUTTER_TTL"=w1390:u8, "TRIGGER_MODE"=w1368:u8, "FRAME_TRANSFER"=w1369:bool, "ACQUISITION_MODE"=w1391:u8, "EM_MODE"=w1359:u8)
                n738 = local read "CH2on"() -> (w1349:bool)
                n739 = case shown="False" w1349 {
                  tunnel: w1388 -> [_ w1429]
                  tunnel: w1387 -> [_ w1428]
                  tunnel: w1386 -> [_ w1427]
                  tunnel: w1385 -> [_ w1426]
                  tunnel: w1384 -> [_ w1425]
                  tunnel: w1383 -> [_ w1424]
                  tunnel: w1382 -> [_ w1423]
                  tunnel: w1381 -> [_ w1422]
                  tunnel: w1380 -> [_ w1421]
                  tunnel: w1379 -> [_ w1420]
                  tunnel: w1378 -> [_ w1419]
                  tunnel: w1377 -> [_ w1418]
                  tunnel: w1376 -> [_ w1417]
                  tunnel: w1375 -> [_ w1416]
                  tunnel: w1374 -> [_ w1415]
                  tunnel: w1373 -> [_ w1414]
                  tunnel: w1372 -> [_ w1413]
                  tunnel: w1371 -> [_ w1412]
                  tunnel: w1347 -> [_ w1411]
                  tunnel: w1346 -> [_ w1410]
                  tunnel: w1370 -> [_ w1409]
                  tunnel: [T12."Disabled and Grayed Out" ("Disabled") T12."Enabled" ("Disabled")] -> w1348
                  frame False {
                    w1407 = FALSE ("Blinking")
                    n740 = property on="Image FInal Column 2" class="DigNum (strict)"("Blinking"=w1407) -> ()  [unwired: 2 in, 2 out]
                    n741 = property on="Frame Transfer 2" class="Bool (strict)"("Blinking"=w1407) -> ()  [unwired: 2 in, 2 out]
                    n742 = property on="Vertical Clock Voltage 2" class="Ring (strict)"("Blinking"=w1407) -> ()  [unwired: 2 in, 2 out]
                    n743 = property on="A/D Channel 2" class="DigNum (strict)"("Blinking"=w1407) -> ()  [unwired: 2 in, 2 out]
                    n744 = property on="Image Initial Line 2" class="DigNum (strict)"("Blinking"=w1407) -> ()  [unwired: 2 in, 2 out]
                    n745 = property on="Image Initial Column 2" class="DigNum (strict)"("Blinking"=w1407) -> ()  [unwired: 2 in, 2 out]
                    n746 = property on="Image Final Line 2" class="DigNum (strict)"("Blinking"=w1407) -> ()  [unwired: 2 in, 2 out]
                    n747 = property on="Shutter Openning Time 2" class="DigNum (strict)"("Blinking"=w1407) -> ()  [unwired: 2 in, 2 out]
                    n748 = property on="Shutter Closing Time 2" class="DigNum (strict)"("Blinking"=w1407) -> ()  [unwired: 2 in, 2 out]
                    n749 = property on="Vertical Binning 2" class="DigNum (strict)"("Blinking"=w1407) -> ()  [unwired: 2 in, 2 out]
                    n750 = property on="Horizontal Binning 2" class="DigNum (strict)"("Blinking"=w1407) -> ()  [unwired: 2 in, 2 out]
                    n751 = property on="CCD EM Gain 2" class="DigNum (strict)"("Blinking"=w1407) -> ()  [unwired: 2 in, 2 out]
                    n752 = property on="Shutter Mode 2" class="Ring (strict)"("Blinking"=w1407) -> ()  [unwired: 2 in, 2 out]
                    n753 = property on="Shutter TTL 2" class="Ring (strict)"("Blinking"=w1407) -> ()  [unwired: 2 in, 2 out]
                    n754 = property on="Acquisition Mode 2" class="Ring (strict)"("Blinking"=w1407) -> ()  [unwired: 2 in, 2 out]
                    n755 = property on="Readout Rate 2" class="Ring (strict)"("Blinking"=w1407) -> ()  [unwired: 2 in, 2 out]
                    n756 = property on="Vertical Shift Speed 2" class="Ring (strict)"("Blinking"=w1407) -> ()  [unwired: 2 in, 2 out]
                    n757 = property on="CCD EM Mode 2" class="Ring (strict)"("Blinking"=w1407) -> ()  [unwired: 2 in, 2 out]
                    n758 = property on="Trigger Mode 2" class="Ring (strict)"("Blinking"=w1407) -> ()  [unwired: 2 in, 2 out]
                    n759 = property on="Read Mode 2" class="Ring (strict)"("Blinking"=w1407) -> ()  [unwired: 2 in, 2 out]
                    n760 = property on="Pre-amplification Gain 2" class="Ring (strict)"("Blinking"=w1407) -> ()  [unwired: 2 in, 2 out]
                  }
                  frame True {
                    n761 = Not(x=w1426) -> (.not. x?=w1447:bool)
                    n762 = Not(x=w1425) -> (.not. x?=w1445:bool)
                    n763 = Not(x=w1424) -> (.not. x?=w1446:bool)
                    n764 = Not(x=w1423) -> (.not. x?=w1444:bool)
                    n765 = Not(x=w1429) -> (.not. x?=w1449:bool)
                    n766 = Not(x=w1428) -> (.not. x?=w1448:bool)
                    n767 = Not(x=w1427) -> (.not. x?=w1450:bool)
                    n768 = property on="Image FInal Column 2" class="DigNum (strict)"("Blinking"=w1447) -> ()  [unwired: 2 in, 2 out]
                    n769 = property on="Frame Transfer 2" class="Bool (strict)"("Blinking"=w1445) -> ()  [unwired: 2 in, 2 out]
                    n770 = property on="Vertical Clock Voltage 2" class="Ring (strict)"("Blinking"=w1446) -> ()  [unwired: 2 in, 2 out]
                    n771 = property on="A/D Channel 2" class="DigNum (strict)"("Blinking"=w1444) -> ()  [unwired: 2 in, 2 out]
                    n772 = property on="Image Initial Line 2" class="DigNum (strict)"("Blinking"=w1449) -> ()  [unwired: 2 in, 2 out]
                    n773 = property on="Image Initial Column 2" class="DigNum (strict)"("Blinking"=w1448) -> ()  [unwired: 2 in, 2 out]
                    n774 = property on="Image Final Line 2" class="DigNum (strict)"("Blinking"=w1450) -> ()  [unwired: 2 in, 2 out]
                    n775 = Not(x=w1419) -> (.not. x?=w1440:bool)
                    n776 = Not(x=w1418) -> (.not. x?=w1442:bool)
                    n777 = Not(x=w1417) -> (.not. x?=w1441:bool)
                    n778 = Not(x=w1416) -> (.not. x?=w1443:bool)
                    n779 = Not(x=w1422) -> (.not. x?=w1438:bool)
                    n780 = Not(x=w1421) -> (.not. x?=w1439:bool)
                    n781 = Not(x=w1420) -> (.not. x?=w1437:bool)
                    n782 = property on="Shutter Openning Time 2" class="DigNum (strict)"("Blinking"=w1440) -> ()  [unwired: 2 in, 2 out]
                    n783 = property on="Shutter Closing Time 2" class="DigNum (strict)"("Blinking"=w1442) -> ()  [unwired: 2 in, 2 out]
